vi "CCM-Check Mandatory Connections.vi"(5 "Tables":cluster{"Table":T1[]}[](array[cluster]), 7 "Mandatory":cluster{"Items":string[]}[](array[cluster]), 11 "error in (no error)":errorcluster) -> (6 "Tables thru":cluster{"Table":T1[]}[](array[cluster]), 15 "error out":errorcluster)   [LabVIEW 2020]
uses:
  Type Defs/CM-Connection.ctl
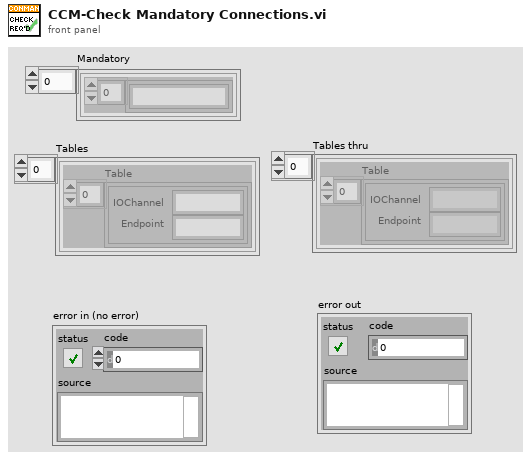
[diagram p1: front panel]
types:
  T1 = typedef "CM-Connection.ctl" = cluster{"IOChannel":string, "Endpoint":string}
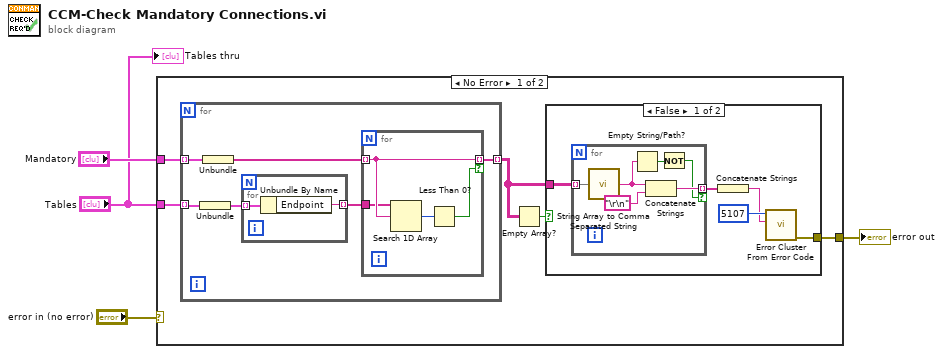
[diagram p0: block diagram]
diagram:
  n1 = case shown="No Error" "error in (no error)" {
    selector: "error in (no error)" -> [_ w33]
    tunnel: [w7 w33] -> w4
    tunnel: "Mandatory" -> [w6 _]
    tunnel: "Tables" -> [w5 _]
    frame No Error {
      n2 = for {
        tunnel: [w15] -> w9 mode=indexing
        tunnel: w6 -> [w13] mode=indexing
        tunnel: w5 -> [w11] mode=indexing
        n3 = Unbundle(w11) -> ("Table"=w10:T1[])
        n4 = Unbundle(w13) -> ("Items"=w12:string[])
        n5 = for {
          tunnel: [w16] -> w14 mode=indexing
          tunnel: w10 -> [w17] mode=indexing
          n6 = Unbundle By Name(w17) -> ("Endpoint"=w16:string)
        }
        n7 = for {
          tunnel: w14 -> [w18]
          tunnel: [w19] -> w15 mode=indexing if=w20
          tunnel: w12 -> [w19] mode=indexing
          n8 = Search 1D Array(1D array=w18, element=w19) -> (index of element=w21:i32)  [unwired: 1 in]
          n9 = Less Than 0?(x=w21) -> (x < 0?=w20:bool)
        }
      }
      n10 = Empty Array?(array=w9) -> (empty?=w8:bool)
      n11 = case shown="False" w8 {
        tunnel: w9 -> [w24 _]
        tunnel: [w25 _] -> w7
        frame False {
          n12 = for {
            tunnel: w24 -> [w31] mode=indexing
            tunnel: [w30] -> w23 mode=indexing if=w29
            n13 = call "String Array to Comma Separated String.vi"("String Array"=w31) -> ("comma separated string"=w27:string)
            n14 = Empty String/Path?(string/path=w27) -> (empty?=w28:bool)
            n15 = Concatenate Strings(w27, "\r\n") -> (w30:string)
            n16 = Not(x=w28) -> (.not. x?=w29:bool)
          }
          n17 = Concatenate Strings(w23) -> (w22:string)
          n18 = call <vilib>:"Error Cluster From Error Code.vi"("error message (\"\")"=w22, "error code (0)"=5107 ("specific error code to clear (0: all)")) -> ("error out"=w25:errorcluster)  [unwired: 7 in]
        }
        frame True {
        }
      }
    }
    frame Error {
    }
  }
  "error out" <- w4
  "Tables thru" <- "Tables"
